vi "freq file read-write controller.vi"(6 "Sweep folder path":path=path "\\\\rus-one\\newdata/data/Ultrasound/Experiment/ProbeTest/Probe10/Hg1201-4-C199-80K-1/Sweep1", 7 "action":T2=enum."init", 8 "Numeric":dbl, 11 "save/read":refnum<vi>) -> (0 "save read out":T1={"write to a file list"=0, "from file "="1827_a", "erase"=FALSE, "load"=FALSE, "save"=FALSE, "to a file "="1827_a", "read from file list"=0} {"read from file list" items=["769_a", "841_a", "1399_a", "1502_a", "1527_a", "1705_a", "1916_a", "1958_a", "2061_a", "2227_a", "2365_a", "2551_a", "2713_a", "2761_a", "2964_a", "3000_a", "3030_a", "3084_a", "3235_a", "3366_a"]}, 1 "Numeric out":dbl, 3 "save/read OUT":refnum<vi>)   [LabVIEW 2021]
uses:
  freq file read-write control.ctl
  save-read action.ctl
  <vilib>/regexp/Match Regular Expression.xnode
panel:
  in  "load":bool caption="read"
  in  "regexp":string="(from file).*"
  in  "read from file list":u16(ring) items=["769_a", "841_a", "1399_a", "1502_a", "1527_a", "1705_a", "1916_a", "1958_a", "2061_a", "2227_a", "2365_a", "2551_a", "2713_a", "2761_a", "2964_a", "3000_a", "3030_a", "3084_a", "3235_a", "3366_a"]
  in  "save/read":T1={"write to a file list"=0, "from file "="1827_a", "erase"=FALSE, "load"=FALSE, "save"=FALSE, "to a file "="1827_a", "read from file list"=0} {"read from file list" items=["2239_a", "2248_a", "2436_a", "2437_a"]; "write to a file list" items=["769_a", "841_a", "1399_a", "1502_a", "1527_a", "1705_a", "1916_a", "1958_a", "2061_a", "2227_a", "2365_a", "2551_a", "2713_a", "2761_a", "2964_a", "3000_a", "3030_a", "3084_a", "3235_a", "3366_a"]}
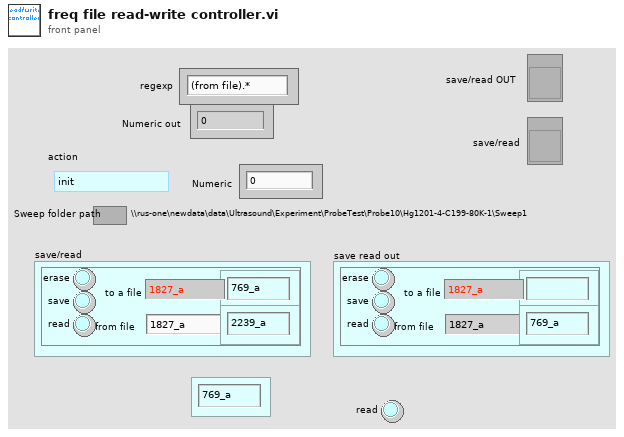
[diagram p1: front panel]
types:
  T1 = typedef "freq file read-write control.ctl" = cluster{"write to a file list":u16, "from file ":string, "erase":bool, "load":bool, "save":bool, "to a file ":string, "read from file list":u16}
  T2 = typedef "save-read action.ctl" = enum16{"update save list", "update read list", "init", "check", "lookup read number", "lookup write number", "copy read from read ring", "saved file dirty", "saved file clean", "read file OK", "read file not OK", "nearest right", "nearest left", "increment read from", "copy read to save", "init save file", "erase event", "save event", "read event", "set save file", "decrement read from"}
  T3 = typedef "slide control.ctl" = cluster{"in slide":bool, "direction":bool, "start ":bool, "stop":bool, "next":bool}
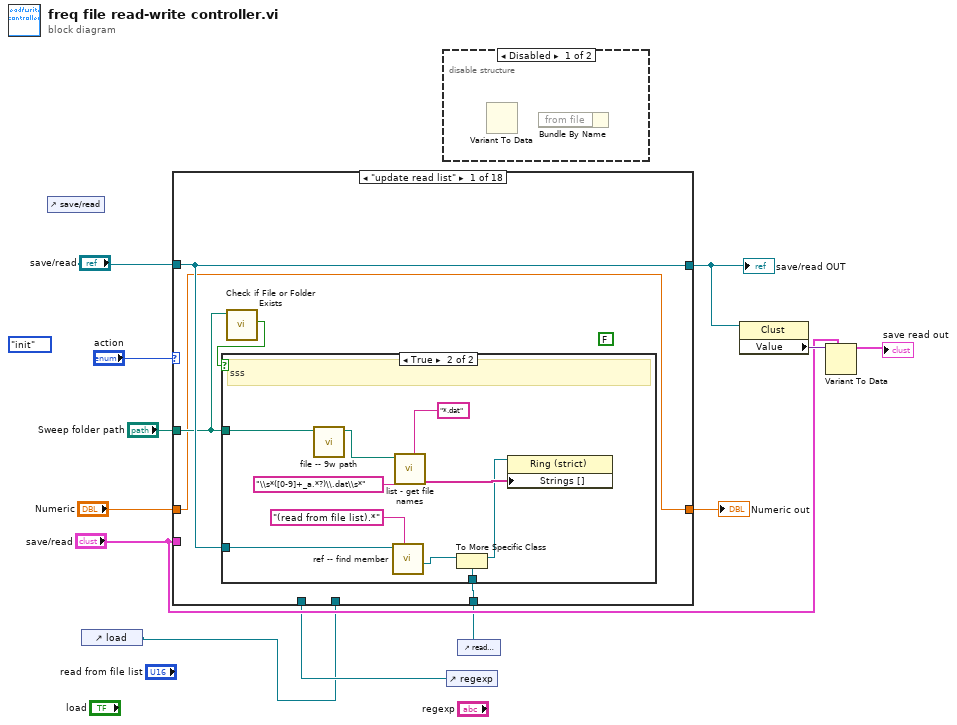
[diagram p0: block diagram]
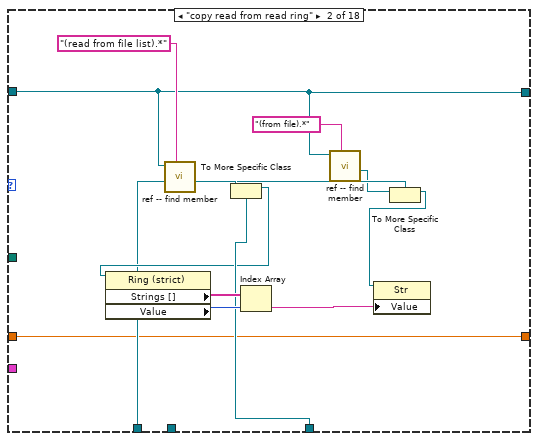
[diagram p4: hidden frame]
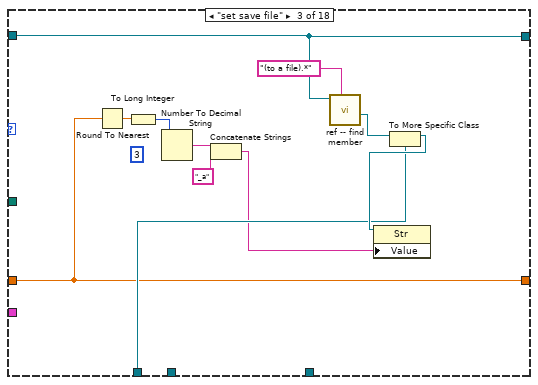
[diagram p5: hidden frame]
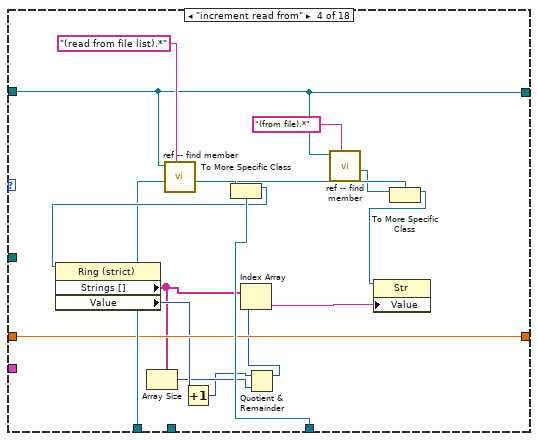
[diagram p6: hidden frame]
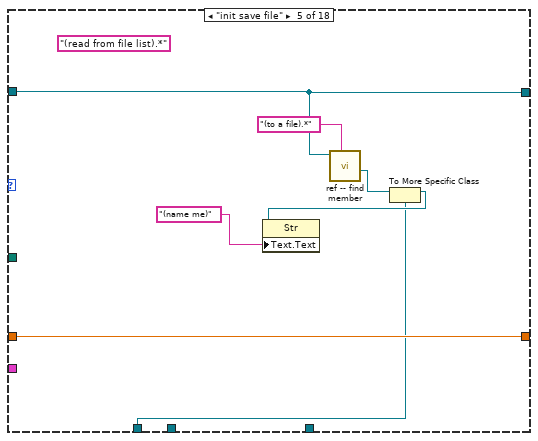
[diagram p7: hidden frame]
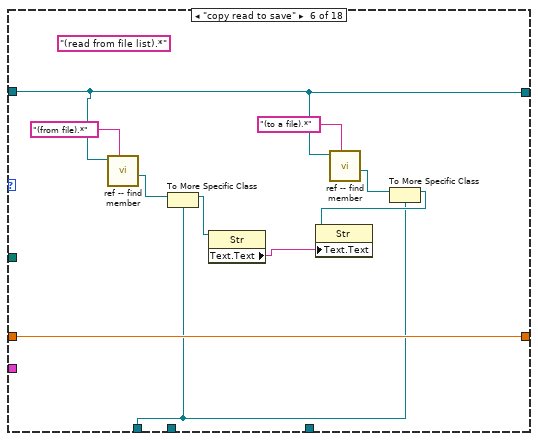
[diagram p8: hidden frame]
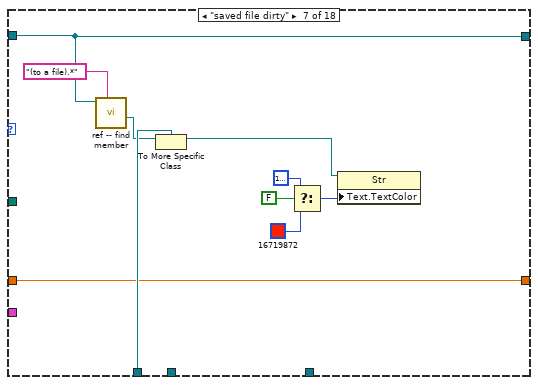
[diagram p9: hidden frame]
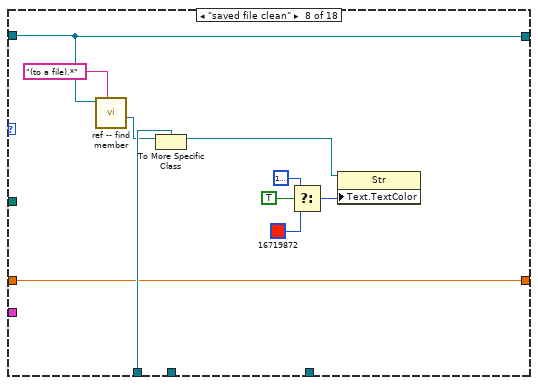
[diagram p10: hidden frame]
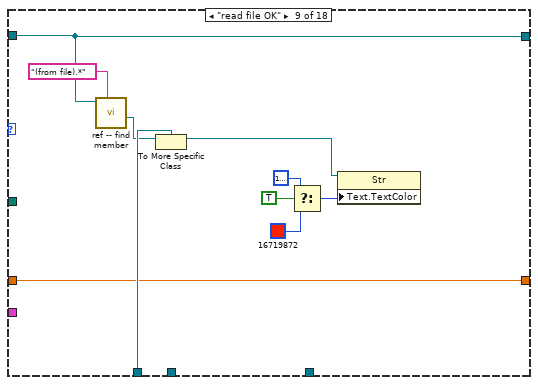
[diagram p11: hidden frame]
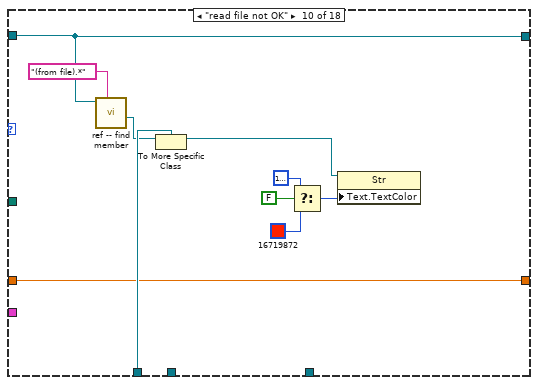
[diagram p12: hidden frame]
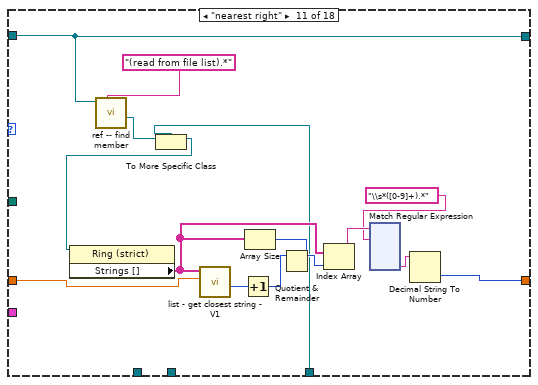
[diagram p13: hidden frame]
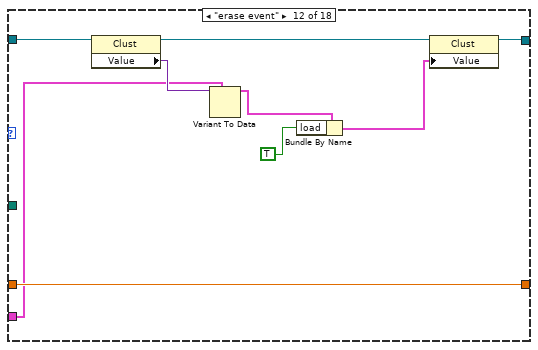
[diagram p14: hidden frame]
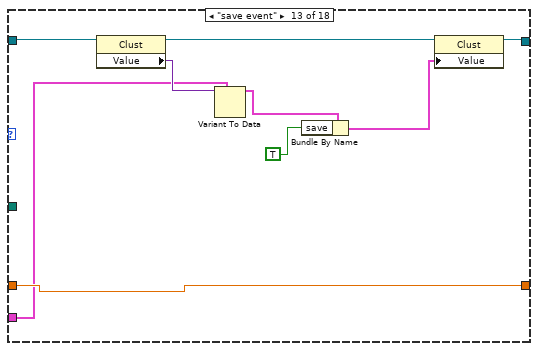
[diagram p15: hidden frame]
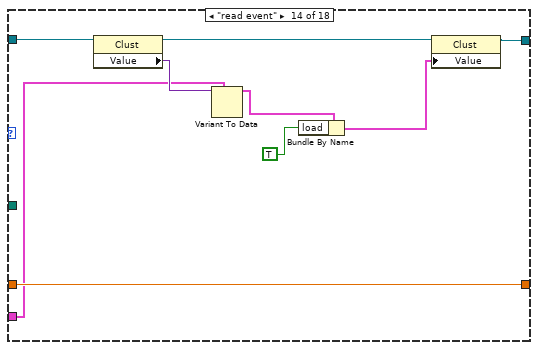
[diagram p16: hidden frame]
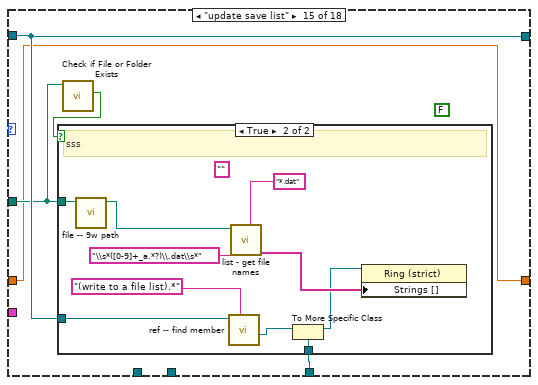
[diagram p17: hidden frame]
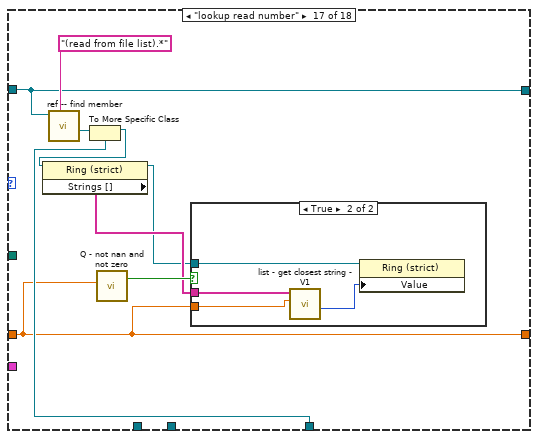
[diagram p20: hidden frame]
diagram:
  (unwired) save-read_action."init" ("action")
  n1 = control-ref of="save/read"() -> ()  [unwired: 1 out]
  n2 = control-ref of="load"() -> (w2:refnum<vi>)
  n3 = disable-structure shown="Disabled" {
    frame Disabled {
      n4 = Variant To Data() -> ()  [unwired: 3 in, 2 out]
      n5 = Bundle By Name() -> ()  [unwired: 2 in, 1 out]
    }
    frame Enabled {
    }
  }
  n6 = control-ref of="regexp"() -> (w4:refnum<vi>)
  n7 = control-ref of="read from file list"() -> (w7:refnum<vi>)
  n8 = case shown="\"update read list\"" "action" {
    tunnel: "save/read" -> [w16 w33 w51 w62 w74 w78 w94 w104 w114 w124 w139 w261 w269 w283 w289 w302 w305 w318]
    tunnel: [w16 w33 w51 w62 w74 w78 w94 w104 w114 w124 w139 w260 w270 w280 w289 w302 w305 w317] -> w12
    tunnel: "save/read" -> [_ _ _ _ _ _ _ _ _ _ _ w259 w268 w282 _ _ _ _]
    tunnel: w7 -> [w17 w35 _ w64 _ _ _ _ _ _ w126 _ _ _ w290 _ w308 _]
    tunnel: "Sweep folder path" -> [w15 _ _ _ _ _ _ _ _ _ _ _ _ _ w288 _ _ _]
    tunnel: "Numeric" -> [w13 w28 w42 w57 w71 w82 w85 w95 w105 w115 w125 w267 w276 w285 w286 w301 w303 w316]
    tunnel: w4 -> [_ w31 w47 w60 w68 w77 w92 w102 w112 w122 _ _ _ _ _ _ _ _]
    tunnel: [w13 w28 w42 w57 w71 w82 w85 w95 w105 w115 w129 w267 w276 w285 w286 w301 w303 w316] -> w3
    tunnel: w2 -> [_ _ _ _ _ _ _ _ _ _ _ _ _ _ _ _ _ _]
    frame "update read list" {
      (unwired) FALSE ("omega ?")
      n9 = call <vilib>:"Check if File or Folder Exists.vi"("path"=w15) -> ("file or folder exists?"=w14:bool)  [unwired: 8 in, 2 out]
      n10 = case shown="True" w14 {
        tunnel: w17 -> [_ w24]
        tunnel: w16 -> [_ w22]
        tunnel: w15 -> [_ w18]
        frame False {
        }
        frame True {
          # "sss"
          n11 = call "file -- 9w path.vi"("sweep folder"=w18) -> ("9w path"=w19:path)  [unwired: 10 in]
          n12 = call "ref -- find member.vi"("regexp"="(read from file list).*", "save/read ref"=w22) -> ("element"=w20:refnum<vi>)  [unwired: 7 in, 2 out]
          n13 = call "list - get file names.vi"("extension filter"="*.dat" ("pattern"), "regular expression"="\\s*([0-9]+_a.*?)\\.dat\\s*", "folder path"=w19) -> ("Array"=w25:string[])  [unwired: 7 in, 1 out]
          n14 = To More Specific Class(target class=w24, reference=w20) -> (specific class reference=w23:refnum<vi>)  [unwired: 1 in, 1 out]
          n15 = property class="Ring (strict)"(reference=w23, "Strings []"=w25) -> ()  [unwired: 1 in, 2 out]
        }
      }
    }
    frame "copy read from read ring" {
      n16 = call "ref -- find member.vi"("regexp"="(read from file list).*", "save/read ref"=w33) -> ("element"=w37:refnum<vi>)  [unwired: 7 in, 2 out]
      n17 = To More Specific Class(target class=w35, reference=w37) -> (specific class reference=w34:refnum<vi>)  [unwired: 1 in, 1 out]
      n18 = property on="Property Node" class="Ring (strict)"(reference=w34) -> ("Strings []"=w40:string[], "Value"=w39:u16)  [unwired: 1 in, 2 out]
      n19 = Index Array(array=w40, index=w39) -> (element=w38:string)
      n20 = call "ref -- find member.vi"("regexp"="(from file).*", "save/read ref"=w33) -> ("element"=w30:refnum<vi>)  [unwired: 7 in, 2 out]
      n21 = To More Specific Class(target class=w31, reference=w30) -> (specific class reference=w29:refnum<vi>)  [unwired: 1 in, 1 out]
      n22 = property on="Property Node" class="Str"(reference=w29, "Value"=w38) -> ()  [unwired: 1 in, 2 out]
    }
    frame "set save file" {
      (unwired) i16 3 ("width (-)")
      n23 = Round To Nearest(number=w42) -> (nearest integer value=w44:dbl)
      n24 = To Long Integer(number=w44) -> (32bit integer=w43:i32)
      n25 = Number To Decimal String(number=w43) -> (decimal integer string=w46:string)  [unwired: 1 in]
      n26 = Concatenate Strings(w46, "_a" ("string")) -> (w41:string)
      n27 = call "ref -- find member.vi"("regexp"="(to a file).*", "save/read ref"=w51) -> ("element"=w49:refnum<vi>)  [unwired: 7 in, 2 out]
      n28 = To More Specific Class(target class=w47, reference=w49) -> (specific class reference=w48:refnum<vi>)  [unwired: 1 in, 1 out]
      n29 = property on="Property Node" class="Str"(reference=w48, "Value"=w41) -> ()  [unwired: 1 in, 2 out]
    }
    frame "increment read from" {
      n30 = call "ref -- find member.vi"("regexp"="(read from file list).*", "save/read ref"=w62) -> ("element"=w66:refnum<vi>)  [unwired: 7 in, 2 out]
      n31 = To More Specific Class(target class=w64, reference=w66) -> (specific class reference=w63:refnum<vi>)  [unwired: 1 in, 1 out]
      n32 = property on="Property Node" class="Ring (strict)"(reference=w63) -> ("Strings []"=w55:string[], "Value"=w56:u16)  [unwired: 1 in, 2 out]
      n33 = Array Size(array=w55) -> (size(s)=w54:i32)
      n34 = Increment(x=w56) -> (x+1=w53:u16)
      n35 = Quotient & Remainder(x=w53, y=w54) -> (x-y*floor(x/y)=w52:i32)  [unwired: 1 out]
      n36 = Index Array(array=w55, index=w52) -> (element=w67:string)
      n37 = call "ref -- find member.vi"("regexp"="(from file).*", "save/read ref"=w62) -> ("element"=w59:refnum<vi>)  [unwired: 7 in, 2 out]
      n38 = To More Specific Class(target class=w60, reference=w59) -> (specific class reference=w58:refnum<vi>)  [unwired: 1 in, 1 out]
      n39 = property on="Property Node" class="Str"(reference=w58, "Value"=w67) -> ()  [unwired: 1 in, 2 out]
    }
    frame "init save file" {
      (unwired) "(read from file list).*" ("regexp")
      n40 = call "ref -- find member.vi"("regexp"="(to a file).*", "save/read ref"=w74) -> ("element"=w72:refnum<vi>)  [unwired: 7 in, 2 out]
      n41 = To More Specific Class(target class=w68, reference=w72) -> (specific class reference=w69:refnum<vi>)  [unwired: 1 in, 1 out]
      n42 = property on="Property Node" class="Str"(reference=w69, "Text.Text"="(name me)") -> ()  [unwired: 1 in, 2 out]
    }
    frame "copy read to save" {
      (unwired) "(read from file list).*" ("regexp")
      n43 = call "ref -- find member.vi"("regexp"="(from file).*", "save/read ref"=w78) -> ("element"=w79:refnum<vi>)  [unwired: 7 in, 2 out]
      n44 = To More Specific Class(target class=w77, reference=w79) -> (specific class reference=w76:refnum<vi>)  [unwired: 1 in, 1 out]
      n45 = property on="Property Node" class="Str"(reference=w76) -> ("Text.Text"=w75:string)  [unwired: 1 in, 2 out]
      n46 = call "ref -- find member.vi"("regexp"="(to a file).*", "save/read ref"=w78) -> ("element"=w83:refnum<vi>)  [unwired: 7 in, 2 out]
      n47 = To More Specific Class(target class=w77, reference=w83) -> (specific class reference=w81:refnum<vi>)  [unwired: 1 in, 1 out]
      n48 = property on="Property Node" class="Str"(reference=w81, "Text.Text"=w75) -> ()  [unwired: 1 in, 2 out]
    }
    frame "saved file dirty" {
      n49 = call "ref -- find member.vi"("regexp"="(to a file).*", "save/read ref"=w94) -> ("element"=w91:refnum<vi>)  [unwired: 7 in, 2 out]
      n50 = To More Specific Class(target class=w92, reference=w91) -> (specific class reference=w87:refnum<vi>)  [unwired: 1 in, 1 out]
      n51 = Select(t=u32 16777222, s=FALSE, f=u32 16719872) -> (s? t:f=w88:u32)
      n52 = property on="Property Node" class="Str"(reference=w87, "Text.TextColor"=w88) -> ()  [unwired: 1 in, 2 out]
    }
    frame "saved file clean" {
      n53 = call "ref -- find member.vi"("regexp"="(to a file).*", "save/read ref"=w104) -> ("element"=w101:refnum<vi>)  [unwired: 7 in, 2 out]
      n54 = To More Specific Class(target class=w102, reference=w101) -> (specific class reference=w97:refnum<vi>)  [unwired: 1 in, 1 out]
      n55 = Select(t=u32 16777222, s=TRUE, f=u32 16719872) -> (s? t:f=w98:u32)
      n56 = property on="Property Node" class="Str"(reference=w97, "Text.TextColor"=w98) -> ()  [unwired: 1 in, 2 out]
    }
    frame "read file OK" {
      n57 = call "ref -- find member.vi"("regexp"="(from file).*", "save/read ref"=w114) -> ("element"=w111:refnum<vi>)  [unwired: 7 in, 2 out]
      n58 = To More Specific Class(target class=w112, reference=w111) -> (specific class reference=w107:refnum<vi>)  [unwired: 1 in, 1 out]
      n59 = Select(t=u32 16777222, s=TRUE, f=u32 16719872) -> (s? t:f=w108:u32)
      n60 = property on="Property Node" class="Str"(reference=w107, "Text.TextColor"=w108) -> ()  [unwired: 1 in, 2 out]
    }
    frame "read file not OK" {
      n61 = call "ref -- find member.vi"("regexp"="(from file).*", "save/read ref"=w124) -> ("element"=w121:refnum<vi>)  [unwired: 7 in, 2 out]
      n62 = To More Specific Class(target class=w122, reference=w121) -> (specific class reference=w117:refnum<vi>)  [unwired: 1 in, 1 out]
      n63 = Select(t=u32 16777222, s=FALSE, f=u32 16719872) -> (s? t:f=w118:u32)
      n64 = property on="Property Node" class="Str"(reference=w117, "Text.TextColor"=w118) -> ()  [unwired: 1 in, 2 out]
    }
    frame "nearest right" {
      n65 = call "ref -- find member.vi"("regexp"="(read from file list).*", "save/read ref"=w139) -> ("element"=w138:refnum<vi>)  [unwired: 7 in, 2 out]
      n66 = To More Specific Class(target class=w126, reference=w138) -> (specific class reference=w127:refnum<vi>)  [unwired: 1 in, 1 out]
      n67 = property class="Ring (strict)"(reference=w127) -> ("Strings []"=w133:string[])  [unwired: 1 in, 2 out]
      n68 = call "list - get closest string - V1.vi"("number"=w125, "string Array"=w133) -> ("closest index"=w137:i32)  [unwired: 7 in, 2 out]
      n69 = Increment(x=w137) -> (x+1=w136:i32)
      n70 = Array Size(array=w133) -> (size(s)=w135:i32)
      n71 = Quotient & Remainder(x=w136, y=w135) -> (x-y*floor(x/y)=w134:i32)  [unwired: 1 out]
      n72 = Index Array(array=w133, index=w134) -> (element=w132:string)
      n73 = xnode "Match Regular Expression"("input string"=w132, "regular expression"="\\s*([0-9]+).*") -> ("submatch 1"=w131:string)  [unwired: 4 in, 5 out]
      n74 = Decimal String To Number(string=w131) -> (number=w129:i32)  [unwired: 2 in, 1 out]
    }
    frame "erase event" {
      n75 = property class="Clust"(reference=w261) -> (reference out=w265:refnum<vi>, "Value"=w266:variant)  [unwired: 1 in, 1 out]
      n76 = Variant To Data(type=w259, Variant=w266) -> (data=w264:T1)  [unwired: 1 in, 1 out]
      n77 = Bundle By Name(cluster=w264, "load"=TRUE ("Value")) -> (w263:T1)
      n78 = property class="Clust"(reference=w265, "Value"=w263) -> (reference out=w260:refnum<vi>)  [unwired: 1 in, 1 out]
    }
    frame "save event" {
      n79 = property class="Clust"(reference=w269) -> (reference out=w274:refnum<vi>, "Value"=w275:variant)  [unwired: 1 in, 1 out]
      n80 = Variant To Data(type=w268, Variant=w275) -> (data=w273:T1)  [unwired: 1 in, 1 out]
      n81 = Bundle By Name(cluster=w273, "save"=TRUE ("Value")) -> (w272:T1)
      n82 = property class="Clust"(reference=w274, "Value"=w272) -> (reference out=w270:refnum<vi>)  [unwired: 1 in, 1 out]
    }
    frame "read event" {
      n83 = property class="Clust"(reference=w283) -> (reference out=w281:refnum<vi>, "Value"=w284:variant)  [unwired: 1 in, 1 out]
      n84 = Variant To Data(type=w282, Variant=w284) -> (data=w279:T1)  [unwired: 1 in, 1 out]
      n85 = Bundle By Name(cluster=w279, "load"=TRUE ("Value")) -> (w278:T1)
      n86 = property class="Clust"(reference=w281, "Value"=w278) -> (reference out=w280:refnum<vi>)  [unwired: 1 in, 1 out]
    }
    frame "update save list" {
      (unwired) FALSE ("omega ?")
      n87 = call <vilib>:"Check if File or Folder Exists.vi"("path"=w288) -> ("file or folder exists?"=w287:bool)  [unwired: 8 in, 2 out]
      n88 = case shown="True" w287 {
        tunnel: w290 -> [_ w297]
        tunnel: w289 -> [_ w295]
        tunnel: w288 -> [_ w292]
        frame False {
        }
        frame True {
          (unwired) "" ("from file")
          # "sss"
          n89 = call "file -- 9w path.vi"("sweep folder"=w292) -> ("9w path"=w293:path)  [unwired: 10 in]
          n90 = call "ref -- find member.vi"("regexp"="(write to a file list).*", "save/read ref"=w295) -> ("element"=w294:refnum<vi>)  [unwired: 7 in, 2 out]
          n91 = call "list - get file names.vi"("extension filter"="*.dat" ("pattern"), "regular expression"="\\s*([0-9]+_a.*?)\\.dat\\s*", "folder path"=w293) -> ("Array"=w298:string[])  [unwired: 7 in, 1 out]
          n92 = To More Specific Class(target class=w297, reference=w294) -> (specific class reference=w296:refnum<vi>)  [unwired: 1 in, 1 out]
          n93 = property class="Ring (strict)"(reference=w296, "Strings []"=w298) -> ()  [unwired: 1 in, 2 out]
        }
      }
    }
    frame "check", Default {
    }
    frame "lookup read number" {
      n94 = call "ref -- find member.vi"("regexp"="(read from file list).*", "save/read ref"=w305) -> ("element"=w309:refnum<vi>)  [unwired: 7 in, 2 out]
      n95 = To More Specific Class(target class=w308, reference=w309) -> (specific class reference=w307:refnum<vi>)  [unwired: 1 in, 1 out]
      n96 = property class="Ring (strict)"(reference=w307) -> (reference out=w304:refnum<vi>, "Strings []"=w306:string[])  [unwired: 1 in, 1 out]
      n97 = call "Q - not nan and not zero.vi"("Numeric"=w303) -> ("Boolean"=w311:bool)  [unwired: 10 in]
      n98 = case shown="True" w311 {
        tunnel: w306 -> [_ w315]
        tunnel: w303 -> [_ w314]
        tunnel: w304 -> [_ w313]
        frame False {
        }
        frame True {
          n99 = call "list - get closest string - V1.vi"("number"=w314, "string Array"=w315) -> ("closest index"=w312:i32)  [unwired: 7 in, 2 out]
          n100 = property class="Ring (strict)"(reference=w313, "Value"=w312) -> ()  [unwired: 1 in, 2 out]
        }
      }
    }
    frame "init" {
      n101 = disable-structure shown="Enabled" {
        disable-tunnel: w318 -> [w323 w325]
        disable-tunnel: [w321 w325] -> w317
        frame Disabled {
          n102 = property class="Clust"(reference=w323) -> (reference out=w322:refnum<vi>, "Value"=w319:variant)  [unwired: 1 in, 1 out]
          n103 = in-place {
            w324 = FALSE ("Boolean")
            n104 = in-place-cluster #1() -> ()  [unwired: 1 in, 5 out]
            n105 = in-place-cluster #1("in slide"=w324, "next"=w324, "direction"=w324, "start"=w324, "stop"=w324) -> (w320:T3)
          }
          n106 = property class="Clust"(reference=w322, "Value"=w320) -> (reference out=w321:refnum<vi>)  [unwired: 1 in, 1 out]
        }
        frame Enabled {
        }
      }
    }
  }
  "Numeric out" <- w3
  "save/read OUT" <- w12
  n107 = property class="Clust"(reference=w12) -> ("Value"=w10:variant)  [unwired: 1 in, 2 out]
  n108 = Variant To Data(type="save/read", Variant=w10) -> (data=→"save read out":T1)  [unwired: 1 in, 1 out]
